vi "Check and Tweak Position.vi"(3 "Mode":T6, 5 "Traverse line In":T3 {"Carrier_2 Q (l/min)" format="%#.2f"; "Row Duration (mins)" format="%#.1f"; "Row No" min=0; "Trace Gas Concentration (%)" min=0.0 format="%#_4f"; "Carrier_1 Q (l/min)" format="%#.4f"; "Start X" format="%#.2f"; "Start Y" format="%#.2f"; "Start Z" format="%#.2f"; "End X" format="%#.2f"; "End Y" format="%#.2f"; "End Z" format="%#.2f"; "Tunnel Speed" format="%#.2f"; "Averaging time (mins)" min=0.0 format="%#.2f"}) -> (0 "Error Message":string, 1 "Status":T2, 2 "Traverse line Out":T3 {"Carrier_2 Q (l/min)" format="%#.2f"; "Row Duration (mins)" format="%#.1f"; "Row No" min=0; "Trace Gas Concentration (%)" min=0.0 format="%#_4f"; "Carrier_1 Q (l/min)" format="%#.4f"; "Start X" format="%#.2f"; "Start Y" format="%#.2f"; "Start Z" format="%#.2f"; "End X" format="%#.2f"; "End Y" format="%#.2f"; "End Z" format="%#.2f"; "Tunnel Speed" format="%#.2f"; "Averaging time (mins)" min=0.0 format="%#.2f"})   [LabVIEW 2022 SP3]
uses:
  Gen Trav/Traverse_cluster.ctl
  Gen Trav/Spacing.ctl
  Controls/Multi_run_mode.ctl
  Controls/User_Specific_mode.ctl
  Gen Trav/Multi_Run_Status.ctl
  Controls/ok_button.ctl
  Globals/Trav_pos_global.vi
panel:
  in  "OK":T1
  in  "stop":bool
  out "Trav Position achieved":sgl[](array[numeric]) format="%#.2f"
  in  "Apply Offset?":bool
  in  "Position Offset":sgl[](array[numeric])=[0.0, 0.0, 0.0] step=1 format="%#.2f"
  # "Happy with Current Position?"
  # "X           Y          Z"
  # "Start"
  # "End"
  # "X           Y          Z"
  # "Start"
  # "End"
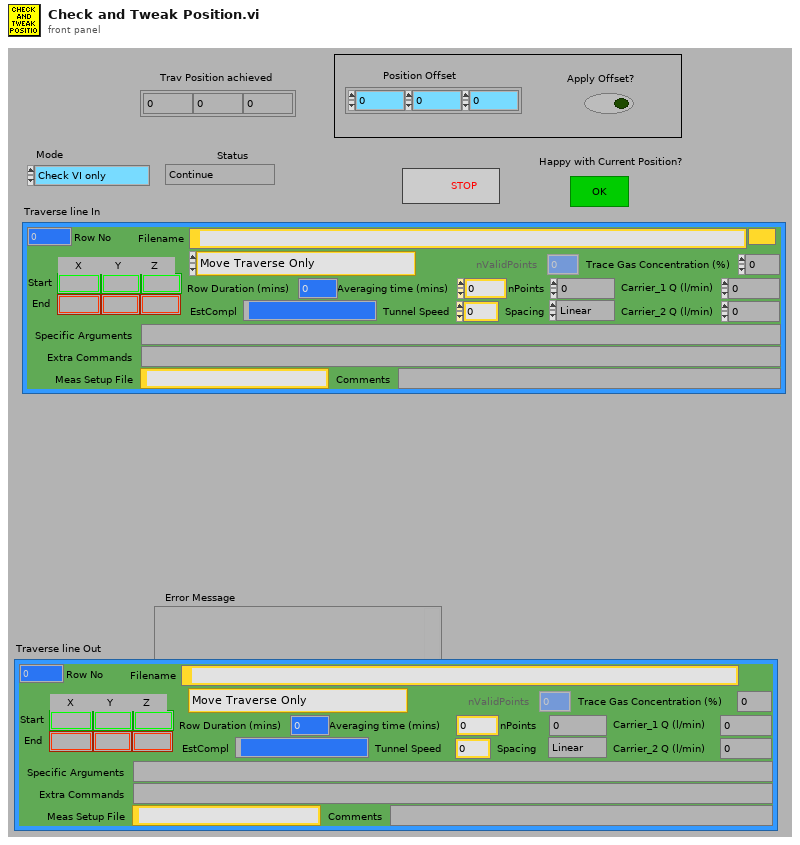
[diagram p1: front panel]
types:
  T1 = typedef "ok_button.ctl" = bool
  T2 = typedef "Multi_Run_Status.ctl" = enum16{"Continue", "Continue with Error", "Jump to Next Point", "Jump to Next Row", "Jump To Fall Back", "Terminate Run"}
  T3 = typedef "Traverse_cluster.ctl" = cluster{"Start X":sgl, "Start Y":sgl, "Start Z":sgl, "End X":sgl, "End Y":sgl, "End Z":sgl, "nPoints":i32, "Spacing":T4, "Filename":path, "Tunnel Speed":dbl, "Averaging time (mins)":dbl, "Extra Commands":string, "Carrier_1 Q (l/min)":dbl, "Carrier_2 Q (l/min)":dbl, "Trace Gas Concentration (%)":dbl, "Specific Arguments":string, "Comments":string, "Row No":i32, "Row Type Selector":T5, "EstCompl":string, "Row Duration (mins)":dbl, "nValidPoints":i32, "Meas Setup File":string}
  T4 = typedef "Spacing.ctl" = enum16{"Linear", "Log", "Gauss", "Specified", "N/A"}
  T5 = typedef "Multi_run_mode.ctl" = enum16{"Move Traverse Only", "Set Tunnel Speed Only", "Set Source Only", "Set Measurement Conditions", "Single Measurement", "Vertical Profile", "Lateral Profile", "Longitudinal Profile", "Multi-Axis Profile", "Explore Volume", "Auto Calibrate", "Meas Fast FID Bkgnd", "Check Beam Power", "Scanning Valve Measurement", "Run VI Named:", "Set ADAM Ch", "Wait (minutes)", "Send Message", "Synchronize With:", "Fall Back to this Row", "Turn Off Row Repeating", "Traverse 3D Volume", "Blank Row", "Jump to Fall Back Row"}
  T6 = typedef "User_Specific_mode.ctl" = enum16{"Check VI only", "Run VI"}
  T7 = typedef "Status_Cluster.ctl" = cluster{"Status":T2, "Error Type":string, "Error Description":string}
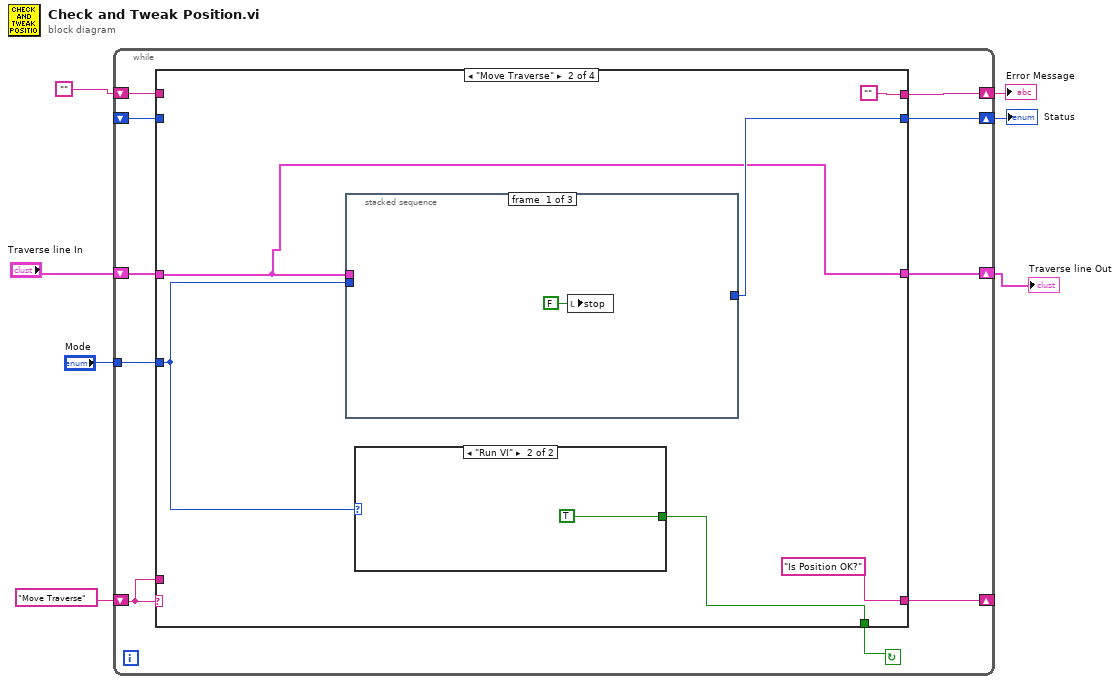
[diagram p0: block diagram]
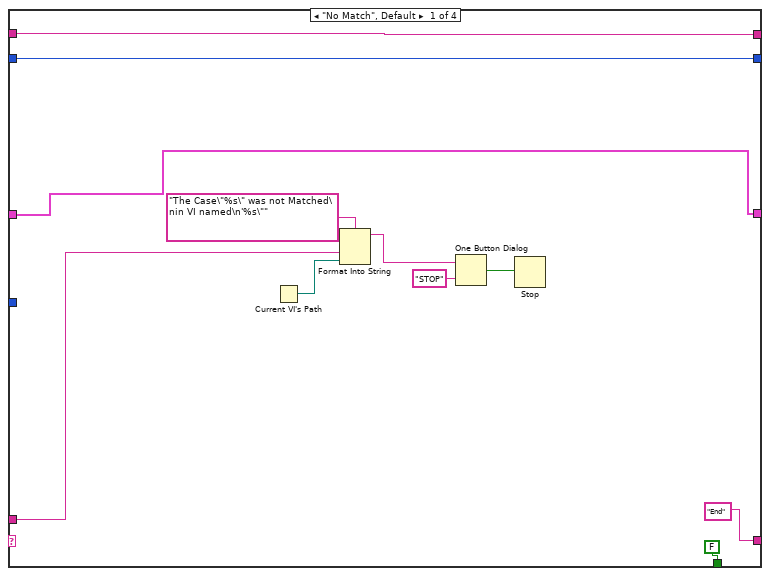
[diagram p2: hidden frame]
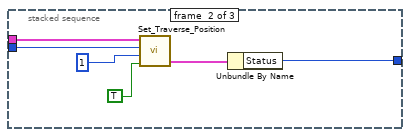
[diagram p3: hidden frame]
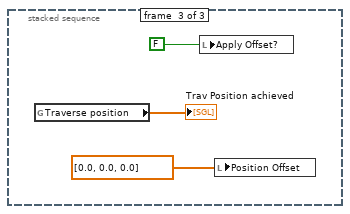
[diagram p4: hidden frame]
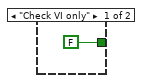
[diagram p5: hidden frame]
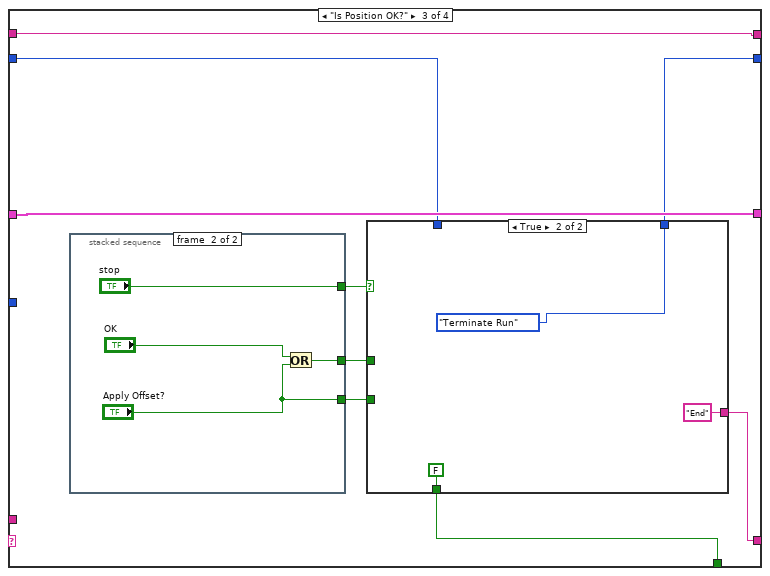
[diagram p6: hidden frame]
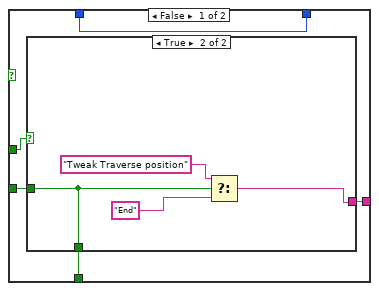
[diagram p7: hidden frame]
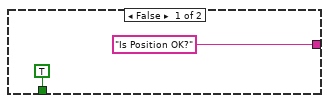
[diagram p8: hidden frame]
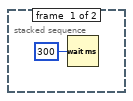
[diagram p9: hidden frame]
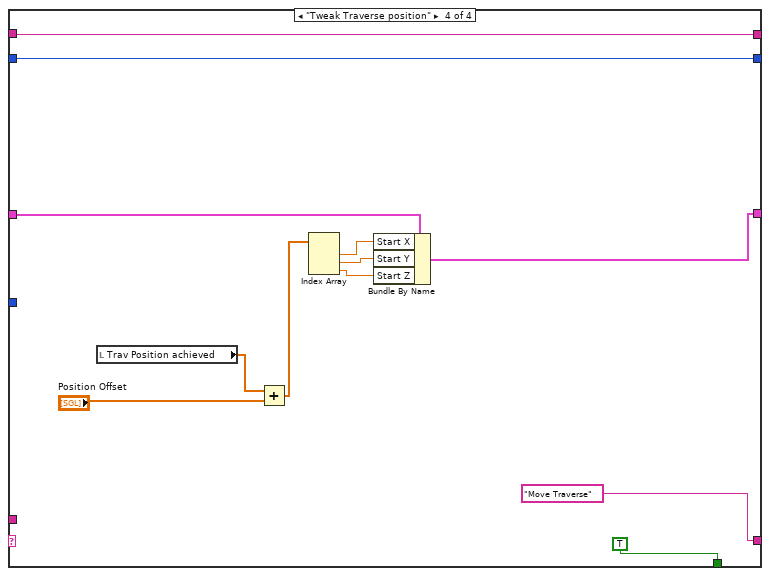
[diagram p10: hidden frame]
diagram:
  n1 = while {
    shift-left: _ -> [w12]
    shift-right: [w11] -> w4
    shift-left: "" -> [w14]
    shift-right: [w13] -> w5
    tunnel: "Mode" -> [w17]
    shift-left: "Move Traverse" -> [w8]
    shift-right: [w15] -> _
    shift-right: [w9] -> w2
    shift-left: "Traverse line In" -> [w10]
    stop <- w16 continue-if-true
    n2 = case shown="\"Move Traverse\"" w8 {
      tunnel: w10 -> [w18 w29 w51 w85]
      tunnel: w17 -> [_ w31 _ _]
      tunnel: [FALSE ("Update Datum Powers?") w33 w50 TRUE ("Tweak Traverse postion")] -> w16
      tunnel: ["End" "Is Position OK?" w53 "Move Traverse"] -> w15
      tunnel: w14 -> [w23 _ w55 w75]
      tunnel: [w23 "" w55 w75] -> w13
      tunnel: w12 -> [w20 _ w47 w76]
      tunnel: [w20 w30 w48 w76] -> w11
      tunnel: [w18 w29 w51 w79] -> w9
      tunnel: w8 -> [w19 _ _ _]
      frame "No Match", Default {
        n3 = Current VI's Path() -> (path=w24:path)
        n4 = Format Into String(format string="The Case\"%s\" was not Matched\nin VI named\n'%s\"" ("Format String"), w19, w24) -> (resulting string=w27:string)  [unwired: 2 in, 1 out]
        n5 = One Button Dialog(message=w27, button name ("OK")="STOP") -> (true=w25:bool)
        n6 = Stop(stop? (T)=w25) -> ()
      }
      frame "Move Traverse" {
        n7 = stacked-sequence {
          tunnel: w29 -> [_ w41 _]
          tunnel: w31 -> [_ w40 _]
          tunnel: [_ w38 _] -> w30
          frame #0 {
            n8 = local write "stop"(FALSE ("stop")) -> ()
          }
          frame #1 {
            n9 = call "Set_Traverse_Position.vi"("Last Part of Move?"=TRUE, "Currently on Point"=1, "Simulate/Run"=w40, "Traverse line"=w41) -> ("Status Cluster"=w39:T7)  [unwired: 2 in]
            n10 = Unbundle By Name(w39) -> ("Status"=w38:T2)
          }
          frame #2 {
            n11 = global read "Trav_pos_global.vi" "Traverse position"() -> (→"Trav Position achieved":sgl[])
            n12 = local write "Apply Offset?"(FALSE ("Tweak Traverse postion")) -> ()
            n13 = local write "Position Offset"(sgl[] [0.0, 0.0, 0.0] ("Position Offset")) -> ()
          }
        }
        n14 = case shown="\"Run VI\"" w31 {
          tunnel: [FALSE ("Update Datum Powers?") TRUE ("Update Datum Powers?")] -> w33
          frame "Check VI only" {
          }
          frame "Run VI" {
          }
        }
      }
      frame "Is Position OK?" {
        n15 = stacked-sequence {
          tunnel: [_ w73] -> w54
          tunnel: [_ "Apply Offset?"] -> w52
          tunnel: [_ "stop"] -> w49
          frame #0 {
            n16 = Wait (ms)(milliseconds to wait=u32 300) -> ()  [unwired: 1 out]
          }
          frame #1 {
            n17 = Or(x="OK", y="Apply Offset?") -> (x .or. y?=w73:T1)
          }
        }
        n18 = case shown="True" w49 {
          tunnel: w54 -> [w60 _]
          tunnel: [w59 "End" ("f")] -> w53
          tunnel: w52 -> [w58 _]
          tunnel: [w57 FALSE ("Tweak Traverse postion")] -> w50
          tunnel: [w56 Multi_Run_Status."Terminate Run" ("Status")] -> w48
          tunnel: w47 -> [w56 _]
          frame False {
            n19 = case shown="True" w60 {
              tunnel: ["Is Position OK?" w64] -> w59
              tunnel: w58 -> [_ w63]
              tunnel: [TRUE ("Tweak Traverse postion") w63] -> w57
              frame False {
              }
              frame True {
                n20 = Select(t="Tweak Traverse position", s=w63, f="End") -> (s? t:f=w64:string)
              }
            }
          }
          frame True {
          }
        }
      }
      frame "Tweak Traverse position" {
        n21 = local read "Trav Position achieved"() -> (w84:sgl[])
        n22 = Add(x=w84, y="Position Offset") -> (x+y=w83:sgl[])
        n23 = Index Array(array=w83) -> (element #1=w82:sgl, element #2=w81:sgl, element #3=w80:sgl)  [unwired: 3 in]
        n24 = Bundle By Name(cluster=w85, "Start X"=w82, "Start Y"=w81, "Start Z"=w80) -> (w79:T3)
      }
    }
  }
  "Status" <- w4
  "Traverse line Out" <- w2
  "Error Message" <- w5
